vi "Configure Multi Eval Meas List Segment Transform Precoding.vi"(5 "Enabled (Off)":bool, 6 "Bandwidth Part (BWP0)":T1 items=["BWP0"], 7 "Carrier Component (1)":T2=1, 8 "error in (no error)":errorcluster, 9 "Segment (1)":T3=1, 10 "Instance (1)":T4=1, 11 "VISA resource name":refnum<visa-resource-name>) -> (0 "error out":errorcluster, 3 "VISA resource name out":refnum<visa-resource-name>)   [LabVIEW 2020, in "Rohde&Schwarz CMXP NR FR2 Measurement.lvlib"]
doc: "Specifies whether the <BWP> on carrier <cc> in segment <no> uses a transform precoding function.\n\nAttribute:\nRSCMXPNRFR2M_ATTR_MULTI_EVAL_MEASUREMENT_LIST_SEGMENT_TRANSFORM_PRECODING\n\nRemote-control command:\nCONFigure:NRMMw:MEAS<i>:LIST:SEGMent<no>[:CC<cc>]:BWPart:PUSCh:DFTPrecoding"
uses:
  <instrlib>/Rohde&Schwarz CMXP NR FR2 Measurement/Rohde&Schwarz CMXP NR FR2 Measurement.lvlib
  <instrlib>/Rohde&Schwarz CMXP NR FR2 Measurement/Private/_Instance.ctl
  <instrlib>/Rohde&Schwarz CMXP NR FR2 Measurement/Private/_Segment.ctl
  <instrlib>/Rohde&Schwarz CMXP NR FR2 Measurement/Private/_Carrier Component.ctl
  <instrlib>/Rohde&Schwarz CMXP NR FR2 Measurement/Private/_Bandwidth Part.ctl
  <instrlib>/Rohde&Schwarz CMXP NR FR2 Measurement/Private/rsidr_core.llb/rsidr_core.lvlib
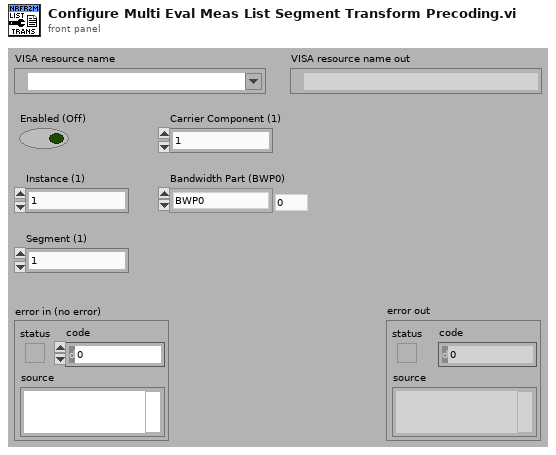
[diagram p1: front panel]
types:
  T1 = typedef "Rohde&Schwarz CMXP NR FR2 Measurement.lvlib/_Bandwidth Part.ctl" = i32
  T2 = typedef "Rohde&Schwarz CMXP NR FR2 Measurement.lvlib/_Carrier Component.ctl" = i32
  T3 = typedef "Rohde&Schwarz CMXP NR FR2 Measurement.lvlib/_Segment.ctl" = i32
  T4 = typedef "Rohde&Schwarz CMXP NR FR2 Measurement.lvlib/_Instance.ctl" = i32
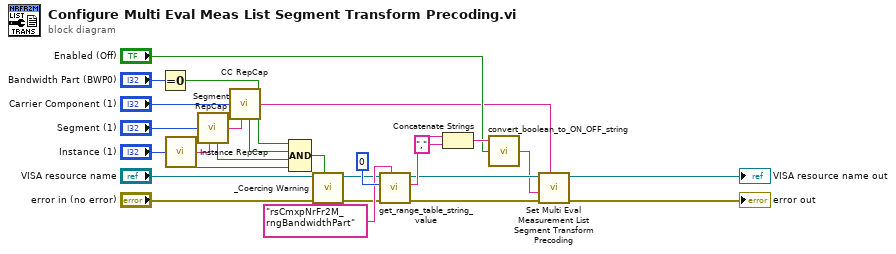
[diagram p0: block diagram]
diagram:
  n1 = Equal To 0?(x="Bandwidth Part (BWP0)") -> (x = 0?=w4:bool)
  n2 = call <instrlib>:"Instance RepCap.vi"("Instance In"="Instance (1)") -> ("In Range?"=w23:bool, "RepCap Identifier Out"=w2:string)  [unwired: 1 in]
  n3 = call <instrlib>:"Segment RepCap.vi"("Segment In"="Segment (1)", "RepCap String In (\"\")"=w2) -> ("In Range?"=w22:bool, "RepCap Identifier Out"=w21:string)
  n4 = call <instrlib>:"CC RepCap.vi"("CC In"="Carrier Component (1)", "RepCap String In (\"\")"=w21) -> ("In Range?"=w20:bool, "RepCap Identifier Out"=w6:string)
  n5 = Compound Arithmetic op=AND(w4, w20, w22, w23) -> (w25:bool)
  n6 = call <instrlib>:"_Coercing Warning.vi"("In Range?"=w25, "error in (no error)"="error in (no error)", "VISA resource name"="VISA resource name") -> ("error out"=w16:errorcluster, "VISA resource name out"=w15:refnum<visa-resource-name>)  [unwired: 7 in]
  n7 = call <instrlib>:"get_range_table_string_value.vi"("Range Table ID in"="rsCmxpNrFr2M_rngBandwidthPart", "error in"=w16, "I32 input"=0, "VISA resource name"=w15) -> ("error out"=w14:errorcluster, "String Value out"=w13:string, "VISA resource name out"=w9:refnum<visa-resource-name>)  [unwired: 5 in]
  n8 = Concatenate Strings(w13, "," ("string")) -> (w11:string)
  n9 = call <instrlib>:"convert_boolean_to_ON_OFF_string.vi"("boolean value in"="Enabled (Off)", "String to add before (\"\")"=w11) -> ("string value out"=w1:string)  [unwired: 3 in]
  n10 = call "Set Multi Eval Measurement List Segment Transform Precoding"("Repeated Capabilities"=w6, "error in (no error)"=w14, "Multi Eval Measurement List Segment Transform Precoding ()"=w1, "instrument handle"=w9) -> ("error out"=→"error out":errorcluster, "instrument handle out"=→"VISA resource name out":refnum<visa-resource-name>)  [unwired: 6 in]
